vi "FV-resample-split_R140_array.vi"(5 "Mid split":i32, 7 "First split":i32, 10 "double array":dbl[](array[numeric])) -> (1 "second subarray":dbl[](array[numeric]), 2 "first subarray":dbl[](array[numeric]))   [LabVIEW 2020, in "FV-file_viewer.lvlib"]
uses:
  FV-file_viewer.lvlib
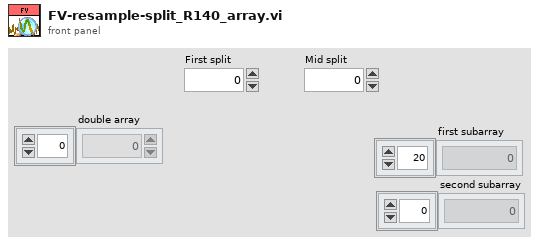
[diagram p1: front panel]
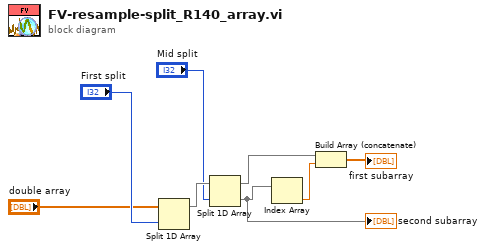
[diagram p0: block diagram]
diagram:
  n1 = Split 1D Array(array="double array", index="First split") -> (first subarray=w8:dbl[])  [unwired: 1 out]
  n2 = Split 1D Array(array=w8, index="Mid split") -> (first subarray=w7:dbl[], second subarray=w6:dbl[])
  "second subarray" <- w6
  n3 = Index Array(array=w6) -> (element=w5:dbl)  [unwired: 1 in]
  n4 = Build Array (concatenate)(w7, w5) -> (→"first subarray":dbl[])
